vi "Auto settings.vi"(8 "error in (no error)":errorcluster, 10 "Array":dbl[](array[numeric]), 11 "Assembly Tray in":refnum<class "Assembly Tray.lvclass">) -> (0 "error out":errorcluster, 3 "Assembly Tray out":refnum<class "Assembly Tray.lvclass">)   [LabVIEW 2020, in "Assembly Tray.lvclass"]
uses:
  Assembly Tray.lvclass
  C:/Users/HEP/Documents/Aerotech gantry/UCSB-Gantry-master-main/V5/Classes/Workspace/Fixture.lvclass
  Assembly Tray.lvclass/Assembly Tray.ctl
  Fixture.lvclass/Fixture.ctl
  Write Gantry Region.vi
  Write Position.vi
  Write Fixture ID.vi
panel:
  in  "Component Thickness":dbl=2.0 format="%#_13g"
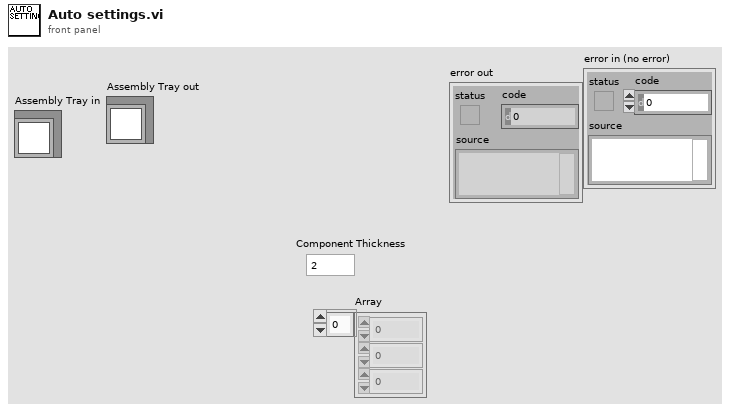
[diagram p1: front panel]
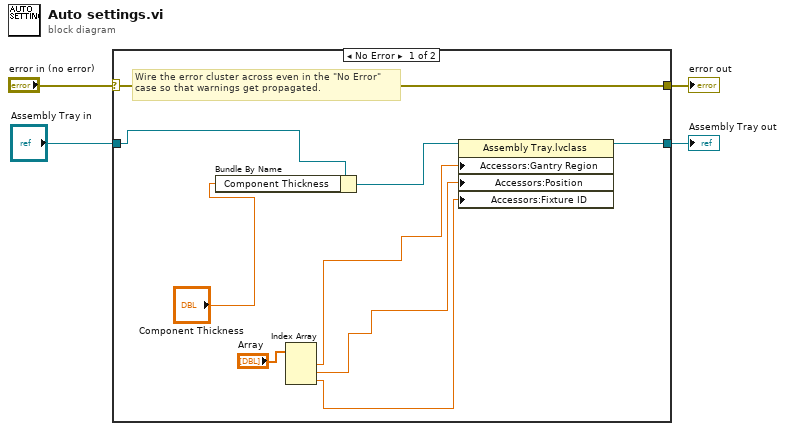
[diagram p0: block diagram]
diagram:
  n1 = case shown="No Error" "error in (no error)" {
    selector: "error in (no error)" -> [w13 w15]
    tunnel: [w13 w15] -> w3
    tunnel: [w12 w14] -> w1
    tunnel: "Assembly Tray in" -> [w11 w14]
    frame No Error {
      # "Wire the error cluster across even in the \"No Error\"\ncase so that warnings get propagated."
      n2 = Bundle By Name(cluster=w11, "Component Thickness"="Component Thickness") -> (w10:refnum<class "Assembly Tray.lvclass">)
      n3 = Index Array(array="Array") -> (element #1=w7:dbl, element #2=w6:dbl, element #3=w5:dbl)  [unwired: 3 in]
      n4 = property class="Assembly Tray.lvclass"(reference=w10, "Accessors:Gantry Region"=w7, "Accessors:Position"=w6, "Accessors:Fixture ID"=w5) -> (reference out=w12:refnum<class "Assembly Tray.lvclass">)  [unwired: 1 in, 1 out]
    }
    frame Error {
    }
  }
  "error out" <- w3
  "Assembly Tray out" <- w1
